vi "Read Pressure Data.vi"(4 "PROM correction Values":u16[](array[numeric]), 6 "I2C Slave Address":u8=119 format="%x", 7 "I2C Channel":u8, 8 "Error In":errorcluster, 10 "dT":i32, 11 "LINX Resource in":T1) -> (0 "Error Out":errorcluster, 1 "Pr mbar":dbl, 3 "LINX Resource out":T1)   [LabVIEW 2014]
uses:
  <vilib>/MakerHub/LINX/Private/Type Defs/LINX Ref.ctl
  <vilib>/MakerHub/LINX/Private/Type Defs/Platform.ctl
  <vilib>/MakerHub/LINX/Private/Type Defs/Interface.ctl
  <vilib>/MakerHub/LINX/Private/Device/Type Defs/LINX Device Config.ctl
  <vilib>/MakerHub/LINX/Private/Device/Type Defs/TCP Config.ctl
  <vilib>/MakerHub/LINX/Private/Device/Type Defs/Channels.ctl
  <vilib>/MakerHub/LINX/Private/Local IO/LinxI2cWrite.vi
  <vilib>/MakerHub/LINX/Public/Utilities/Check Channel.vi
  <vilib>/MakerHub/LINX/Private/Utilties/Generate Error.vi
  <vilib>/MakerHub/LINX/LMH-LINX.lvlib
  <vilib>/MakerHub/LINX/Private/Device/Device.lvlib
panel:
  out "SENS":i64
  out "OFF":i64
  out "C4":u16
  out "C3":u16
  out "C2":u16
  out "C1":u16
  out "D1":u32
  out "D2 Raw Data Values":u16[](array[numeric])
  # "Functional Partameters"
  # "Calculation & Data Results"
  # "Data 23-16"
  # "Data 8-15"
  # "PROM Array Input"
  # "Datas 0-7"
  # "Pressure Correction Factors"
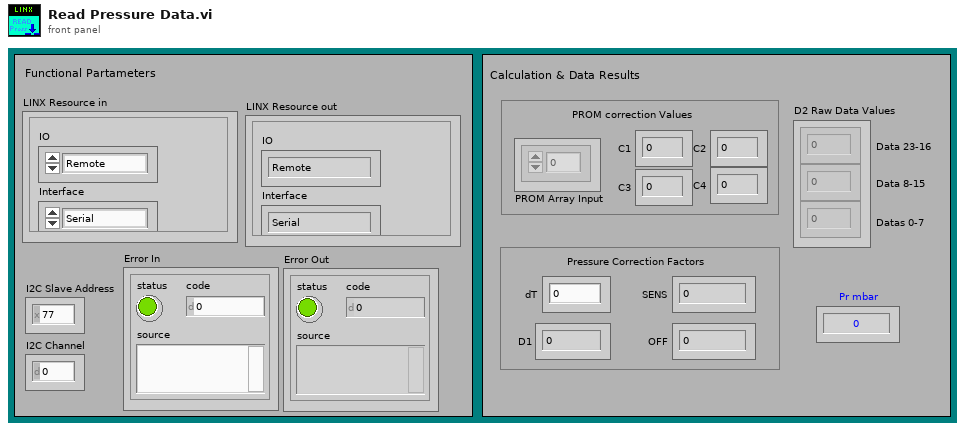
[diagram p1: front panel]
types:
  T1 = typedef "LMH-LINX.lvlib/LINX Ref.ctl" = cluster{"IO":T2, "Interface":T3, "LINX Device Config":T4}
  T2 = typedef "LMH-LINX.lvlib/Platform.ctl" = enum16{"Remote", "Local"}
  T3 = typedef "LMH-LINX.lvlib/Interface.ctl" = enum16{"Serial", "TCP"}
  T4 = typedef "LMH-LINX.lvlib/Device.lvlib/LINX Device Config.ctl" = cluster{"Interface":T3, "COM Port":refnum<visa-resource-name>, "TCP Configuration":T5, "Device Family":u8, "Device ID":u8, "Device Name":string, "TCP Ref":refnum<k5>, "Channels":T6}
  T5 = typedef "LMH-LINX.lvlib/Device.lvlib/TCP Config.ctl" = cluster{"IP Address":string, "Port":u16}
  T6 = typedef "LMH-LINX.lvlib/Channels.ctl" = cluster{"DI":u8[], "DO":u8[], "AI":u8[], "AO":u8[], "PWM":u8[], "QE":u8[], "UART":u8[], "I2C 2":u8[], "SPI":u8[], "CAN":u8[], "Servo":u8[], "AI Ref (V)":dbl, "AI Resolution (Bits)":u8, "AO Ref (V)":dbl, "AO Resolution (Bits)":u8}
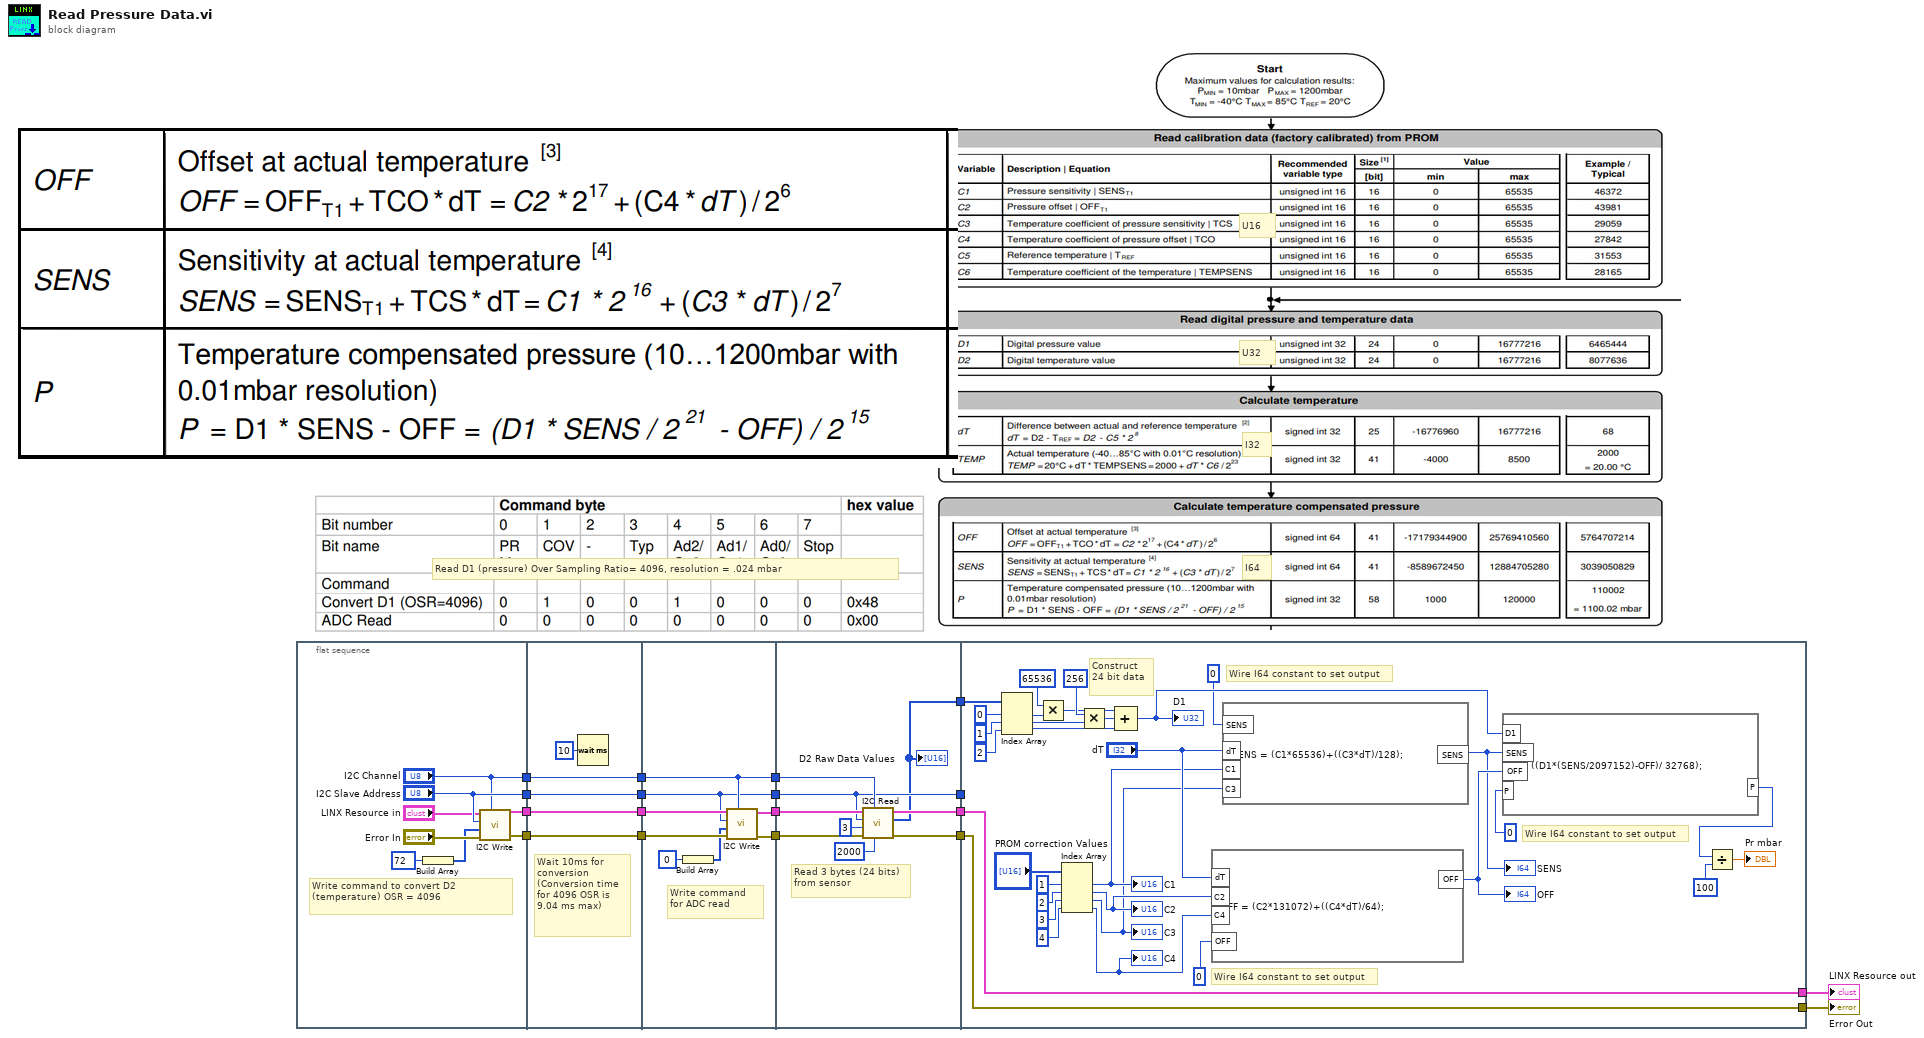
[diagram p0: block diagram]
diagram:
  # "U16"
  # "U32"
  # "I64"
  # "I32"
  # "Read D1 (pressure) Over Sampling Ratio= 4096, resolution = .024 mbar"
  n1 = flat-sequence {
    tunnel: ["I2C Slave Address"] -> w18
    tunnel: ["I2C Channel"] -> w17
    tunnel: [w24] -> w16
    tunnel: [w23] -> w15
    tunnel: w18 -> [w31]
    tunnel: w17 -> [w30]
    tunnel: w16 -> [w29]
    tunnel: w15 -> [w28]
    tunnel: [w31] -> w12
    tunnel: [w30] -> w10
    tunnel: [w29] -> w8
    tunnel: [w28] -> w6
    tunnel: w12 -> [w34]
    tunnel: [w34] -> w11
    tunnel: w10 -> [w35]
    tunnel: [w35] -> w9
    tunnel: w8 -> [w39]
    tunnel: [w37] -> w7
    tunnel: w6 -> [w38]
    tunnel: [w36] -> w5
    tunnel: w11 -> [w41]
    tunnel: w9 -> [w46]
    tunnel: w7 -> [w45]
    tunnel: w5 -> [w44]
    tunnel: [w41] -> w4
    tunnel: [w43] -> w3
    tunnel: [w42] -> w2
    tunnel: [w40] -> w1
    tunnel: [w79] -> w13
    tunnel: [w80] -> w14
    tunnel: w4 -> [_]
    tunnel: w3 -> [w80]
    tunnel: w2 -> [w79]
    tunnel: w1 -> [w78]
    frame #0 {
      # "Write command to convert D2 (temperature) OSR = 4096"
      n2 = Build Array(u8 72) -> (w20:u8[])
      n3 = call <vilib>:"I2C Write.vi"("I2C Channel"="I2C Channel", "Error In"="Error In", "Data"=w20, "I2C Slave Address (0)"="I2C Slave Address", "LINX Resource"="LINX Resource in") -> ("Error Out"=w23:errorcluster, "LINX Resource"=w24:T1)  [unwired: 5 in]
    }
    frame #1 {
      # "Wait 10ms for conversion (Conversion time for 4096 OSR is 9.04 ms max)"
      n4 = Wait (ms)(milliseconds to wait=u32 10) -> ()  [unwired: 1 out]
    }
    frame #2 {
      # "Write command for ADC read"
      n5 = Build Array(u8 0) -> (w32:u8[])
      n6 = call <vilib>:"I2C Write.vi"("I2C Channel"=w35, "Error In"=w38, "Data"=w32, "I2C Slave Address (0)"=w34, "LINX Resource"=w39) -> ("Error Out"=w36:errorcluster, "LINX Resource"=w37:T1)  [unwired: 5 in]
    }
    frame #3 {
      # "Read 3 bytes (24 bits) from sensor"
      n7 = call <vilib>:"I2C Read.vi"("Timeout (1000 ms)"=u16 2000, "I2C Channel"=w46, "Error In"=w44, "Bytes To Read"=u8 3, "I2C Slave Address (0)"=w41, "LINX Resource"=w45) -> ("Error Out"=w43:errorcluster, "Data"=w40:u8[], "LINX Resource"=w42:T1)  [unwired: 3 in]
      "D2 Raw Data Values" <- w40
    }
    frame #4 {
      # "2^15"
      # "2^21"
      # "Wire I64 constant to set output"
      # "Wire I64 constant to set output"
      # "Wire I64 constant to set output"
      # "2^6"
      # "2^16"
      # "2^6"
      # "2^17"
      # "Construct 24 bit data"
      n8 = Index Array(array=w78, index #1=0 ("index"), index #2=1 ("index"), index #3=2 ("index")) -> (element #1=w73:u8, element #2=w70:u8, element #3=w67:u8)
      n9 = Multiply(x=u32 65536 ("y"), y=w73) -> (x*y=w68:u32)
      n10 = Index Array(array="PROM correction Values", index #1=1 ("index"), index #2=2 ("index"), index #3=3 ("index"), index #4=4 ("index")) -> (element #1=w59:u16, element #2=w61:u16, element #3=w58:u16, element #4=w62:u16)
      "C1" <- w59
      "C2" <- w61
      "C3" <- w58
      "C4" <- w62
      n11 = Multiply(x=u32 256 ("y"), y=w70) -> (x*y=w69:u32)
      n12 = Compound Arithmetic op=ADD(w68, w69, w67) -> (w57:u32)
      "D1" <- w57
      n13 = formula code="OFF = (C2*131072)+((C4*dT)/64);"("dT"="dT", "C2"=w61, "C4"=w62, "OFF"=i64 0 ("input variable")) -> ("OFF"=w56:i64)
      "OFF" <- w56
      n14 = formula code="SENS = (C1*65536)+((C3*dT)/128);"("dT"="dT", "C1"=w59, "C3"=w58, "SENS"=i64 0 ("input variable")) -> ("SENS"=w55:i64)
      "SENS" <- w55
      n15 = formula code="P = ((D1*(SENS/2097152)-OFF)/ 32768);"("D1"=w57, "SENS"=w55, "OFF"=w56, "P"=i64 0 ("input variable")) -> ("P"=w51:i64)
      n16 = Divide(x=w51, y=i64 100) -> (x/y=→"Pr mbar":dbl)
    }
  }
  "LINX Resource out" <- w13
  "Error Out" <- w14
